vi "Stellglied - Kopie.vi"(8 "error in (no error)":errorcluster caption="Fehler (Eingang, kein Fehler)", 10 "Stellgröße - Kraft (N)":dbl, 11 "RPDO2 object in":refnum<k20>) -> (0 "error out":errorcluster caption="Fehler (Ausgang)", 3 "Kraft (N)":dbl)   [LabVIEW 2014]
uses:
  <vilib>/CANopenLib/CANOPEN.llb/CANopen Convert To Data [I16].vi
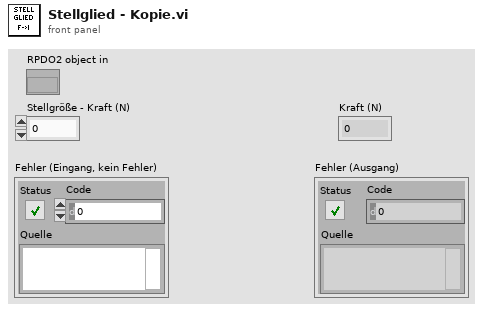
[diagram p1: front panel]
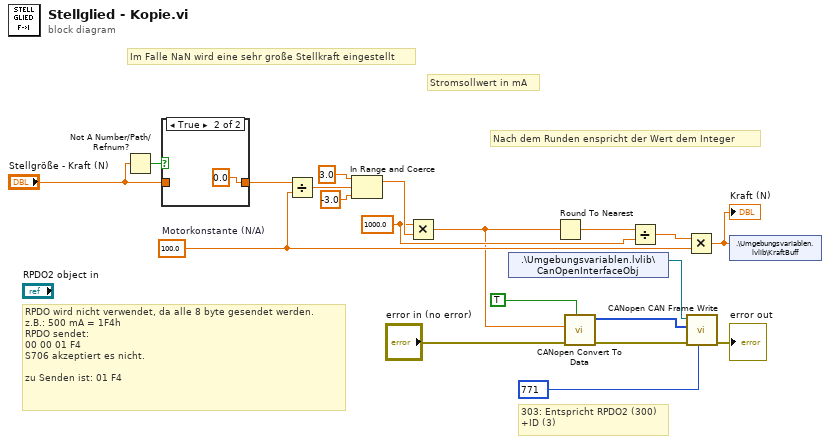
[diagram p0: block diagram]
diagram:
  w14 = 1000.0 ("x")
  w12 = 100.0  # Motorkonstante (N/A)
  # "Im Falle NaN wird eine sehr große Stellkraft eingestellt"
  # "Nach dem Runden enspricht der Wert dem Integer"
  # "RPDO wird nicht verwendet, da alle 8 byte gesendet werden. \nz.B.: 500 mA = 1F4h\nRPDO sendet:\n00 00 01 F4 \nS706 akzeptiert es nicht.\n\nzu Senden ist: 01 F4"
  # "303: Entspricht RPDO2 (300)\n+ID (3)"
  # "Stromsollwert in mA"
  n1 = Not A Number/Path/Refnum?(number/path/refnum="Stellgröße - Kraft (N)") -> (NaN/Path/Refnum?=w7:bool)
  n2 = case shown="True" w7 {
    tunnel: [w21 0.0 ("Stellgröße - Kraft (N)")] -> w5
    tunnel: "Stellgröße - Kraft (N)" -> [w21 _]
    frame False {
    }
    frame True {
    }
  }
  n3 = Divide(x=w5, y=w12) -> (x/y=w16:dbl)
  n4 = In Range and Coerce(upper limit=3.0 ("Obergrenze"), x=w16, lower limit=-3.0 ("Untergrenze")) -> (coerced(x)=w15:dbl)  [unwired: 1 out]
  n5 = Multiply(x=w14, y=w15) -> (x*y=w4:dbl)
  n6 = shared-variable ".\\Umgebungsvariablen.lvlib\\CanOpenInterfaceObj"() -> (w10:refnum<k20>)  [unwired: 1 in, 1 out]
  n7 = Round To Nearest(number=w4) -> (nearest integer value=w2:dbl)
  n8 = call-poly <vilib>:"CANopen Convert To Data.vi"("trim"=TRUE, "error in (no error)"="error in (no error)", "signed 16-bit integer"=w4) -> ("error out"=w9:errorcluster, "CANopen data out"=w3:u8[])  [unwired: 7 in]
  n9 = Divide(x=w2, y=w14) -> (x/y=w13:dbl)
  n10 = Multiply(x=w13, y=w12) -> (x*y=w1:dbl)
  "Kraft (N)" <- w1
  n11 = call <vilib>:"CANopen CAN Frame Write.vi"("COB-ID (0)"=u32 771, "error in (no error)"=w9, "CAN message data"=w3, "interface object  in"=w10) -> ("error out"=→"error out":errorcluster)  [unwired: 6 in, 1 out]
  n12 = shared-variable ".\\Umgebungsvariablen.lvlib\\KraftBuff"(w1) -> ()  [unwired: 1 in, 1 out]
